vi "AVI Video-Close files.vi"(8 "error in (no error)":errorcluster) -> (0 "error out (pass through)":errorcluster)   [LabVIEW 2013]
uses:
  Typedefs/Channel Selector.ctl
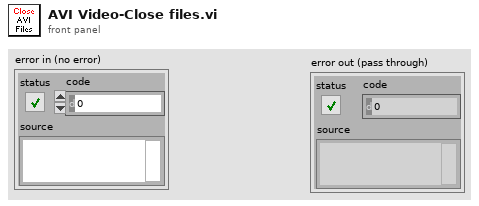
[diagram p1: front panel]
types:
  T1 = typedef "Channel Selector.ctl" = enum16{"Red Channel", "Green Channel", "Blended"}
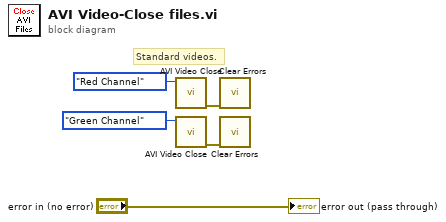
[diagram p0: block diagram]
diagram:
  # "Standard videos."
  n1 = call "AVI Video Close.vi"("Channel"=Channel_Selector."Red Channel") -> ("error out"=w4:errorcluster)  [unwired: 10 in]
  n2 = call "AVI Video Close.vi"("Channel"=Channel_Selector."Green Channel") -> ("error out"=w5:errorcluster)  [unwired: 10 in]
  n3 = call <vilib>:"Clear Errors.vi"("error in (no error)"=w4) -> ()  [unwired: 6 in, 1 out]
  n4 = call <vilib>:"Clear Errors.vi"("error in (no error)"=w5) -> ()  [unwired: 6 in, 1 out]
  "error out (pass through)" <- "error in (no error)"
